vi "Запись 2D массива строк в файл.vi"(2 "путь к файлу":path, 8 "2-D массив строк для записи":string[][](table)) -> ()   [LabVIEW 2013]
uses:
  <vilib>/Utility/file.llb/Write To Spreadsheet File (string).vi
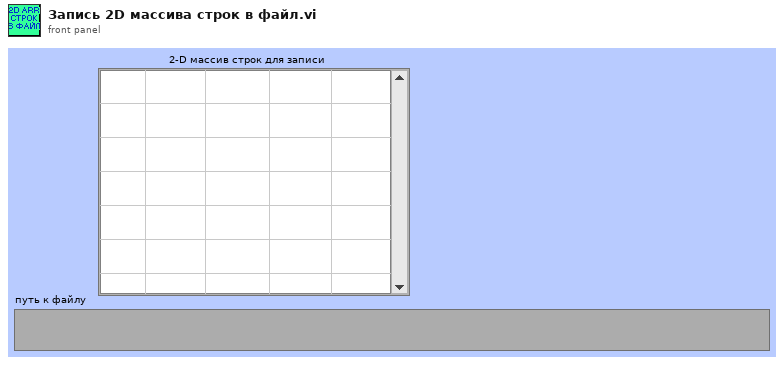
[diagram p1: front panel]
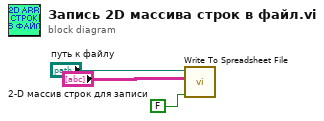
[diagram p0: block diagram]
diagram:
  n1 = call-poly <vilib>:"Write To Spreadsheet File.vi"("append to file? (new file:F)"=FALSE, "2D data"="2-D массив строк для записи", "file path (dialog if empty)"="путь к файлу") -> ()  [unwired: 3 in, 3 out]
